vi "InitializeQGStageOutputChannels.vi"(1 "1st Axis":u16(ring) items=["x", "y"]) -> (0 "Append Channels":tag)   [LabVIEW 2009]
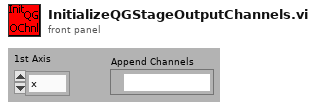
[diagram p1: front panel]
types:
  T1 = typedef "QGSettings.ctt" = cluster{"channels (trigger)":tag, "Trigger Amplitude (V)":dbl}
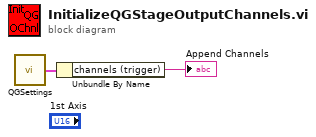
[diagram p0: block diagram]
diagram:
  n1 = call "QGSettings.vi"() -> ("QG Settings (output)"=w2:T1)  [unwired: 2 in]
  n2 = Unbundle By Name(w2) -> ("channels (trigger)"=→"Append Channels":tag)
